vi "Read CCD Config.vi"(8 "error in (no error)":errorcluster, 11 "JSON reader in":refnum<class "JSON reader.lvclass">) -> (0 "error out":errorcluster, 2 "CCD Config":T1, 3 "JSON reader out":refnum<class "JSON reader.lvclass">)   [LabVIEW 2018, in "JSON reader.lvclass"]
uses:
  JSON reader.lvclass
  JSON reader.lvclass/JSON reader.ctl
  Interface/Interface.lvclass
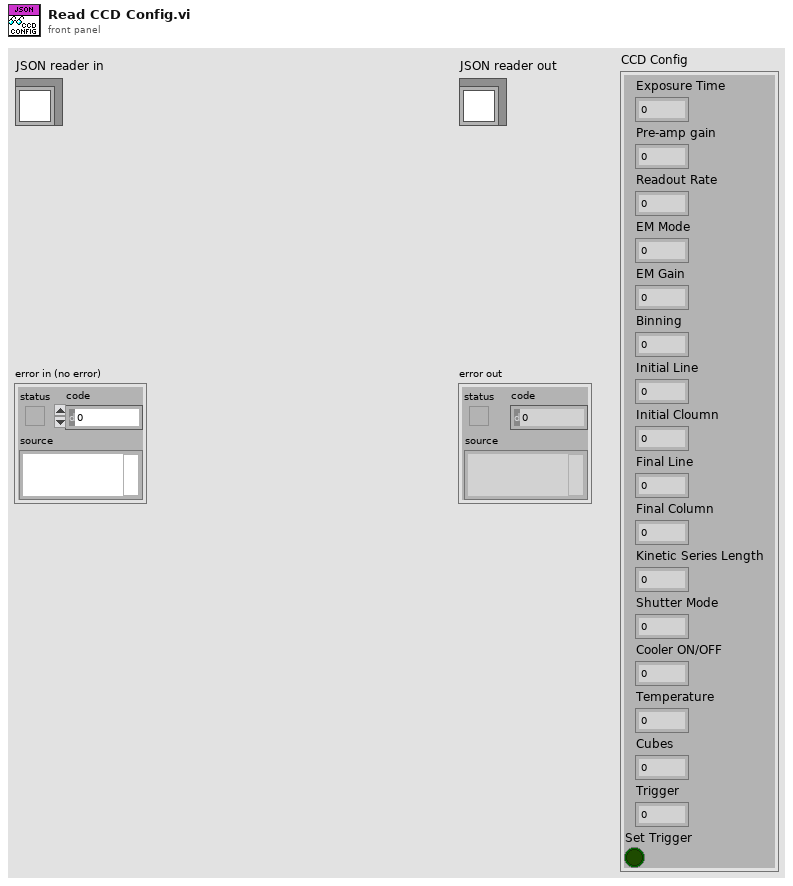
[diagram p1: front panel]
types:
  T1 = cluster{"Exposure Time":sgl, "Pre-amp gain":u8, "Readout Rate":u8, "EM Mode":u8, "EM Gain":u16, "Binning":u16, "Initial Line":u16, "Initial Cloumn":u16, "Final Line":u16, "Final Column":u16, "Kinetic Series Length":u32, "Shutter Mode":u8, "Cooler ON/OFF":u16, "Temperature":i8, "Cubes":u32, "Trigger":u16, "Set Trigger":bool}
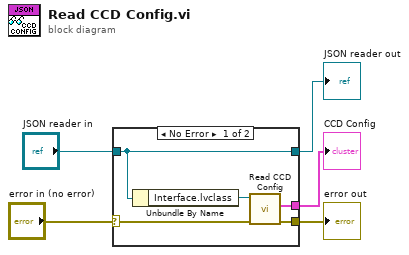
[diagram p0: block diagram]
diagram:
  n1 = case shown="No Error" "error in (no error)" {
    selector: "error in (no error)" -> [w8 w11]
    tunnel: [w9 w11] -> w4
    tunnel: [w10 w12] -> w2
    tunnel: "JSON reader in" -> [w10 w12]
    tunnel: [w6 _] -> w1
    frame No Error {
      n2 = Unbundle By Name(w10) -> ("Interface.lvclass"=w7:refnum<class "Interface.lvclass">)
      n3 = call "Read CCD Config.vi"("error in (no error)"=w8, "Interface in"=w7) -> ("error out"=w9:errorcluster, "CCD Config"=w6:T1)  [unwired: 7 in, 1 out]
    }
    frame Error {
    }
  }
  "error out" <- w4
  "JSON reader out" <- w2
  "CCD Config" <- w1
